vi "Initialize.vi"(8 "Error In":errorcluster, 9 "Buoy Pass 2":T1 {"North" format="%#_10f"; "East" format="%#_8f"}, 10 "Buoy Pass 1":T1 {"North" format="%#_10f"; "East" format="%#_8f"}) -> (0 "Error Out":errorcluster, 3 "PassBuoys out":refnum<class "PassBuoys.lvclass">)   [LabVIEW 2011, in "PassBuoys.lvclass"]
uses:
  PassBuoys.lvclass
  2 Typedefs/UTM Location.ctl
  PassBuoys.lvclass/PassBuoys.ctl
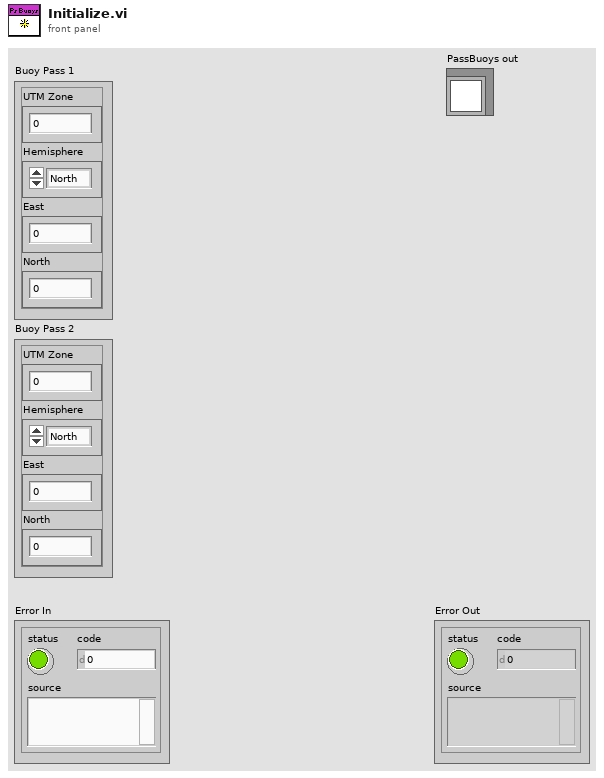
[diagram p1: front panel]
types:
  T1 = typedef "UTM Location.ctl" = cluster{"UTM Zone":dbl, "Hemisphere":enum16{"North", "South"}, "East":dbl, "North":dbl}
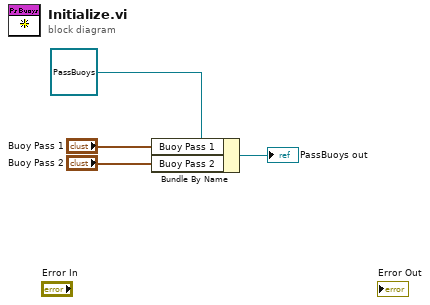
[diagram p0: block diagram]
diagram:
  n1 = Bundle By Name(cluster=refnum<class "PassBuoys.lvclass"> refnum ("PassBuoys in"), "Buoy Pass 1"="Buoy Pass 1", "Buoy Pass 2"="Buoy Pass 2") -> (→"PassBuoys out":refnum<class "PassBuoys.lvclass">)
